vi "Read Tags.vi"(8 "error in (no error)":errorcluster, 11 "Raw Message in":refnum<class "Raw Message.lvclass">) -> (0 "error out":errorcluster, 2 "Tags":map{u32, refnum<class "Basic Type.lvclass">[]}(c390), 3 "Raw Message out":refnum<class "Raw Message.lvclass">)   [LabVIEW 2020, in "Protobuf RAW.lvlib" / "Raw Message.lvclass"]
uses:
  Raw Message.lvclass
  Tag/Basic Type.lvclass
  Raw Message.lvclass/Raw Message.ctl
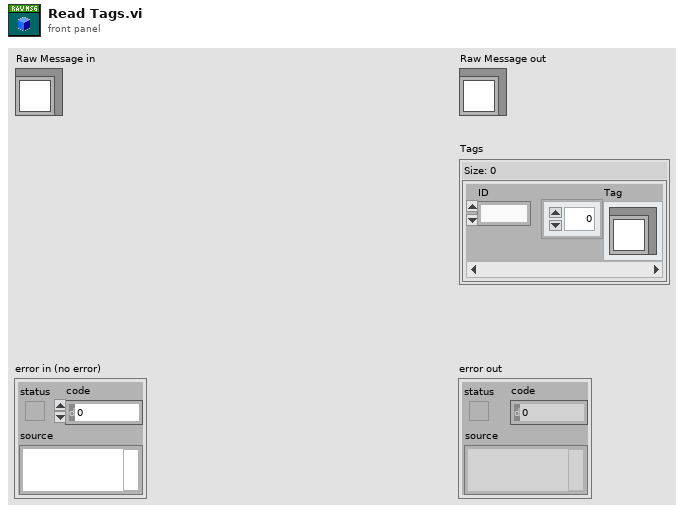
[diagram p1: front panel]
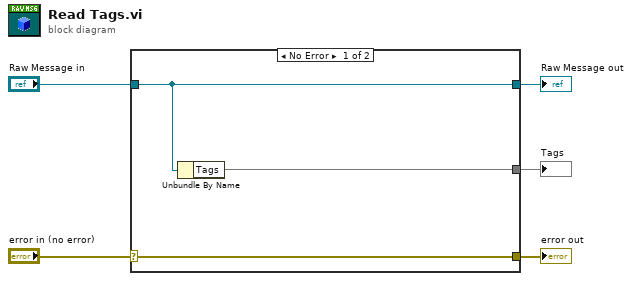
[diagram p0: block diagram]
diagram:
  n1 = case shown="No Error" "error in (no error)" {
    selector: "error in (no error)" -> [w8 w9]
    tunnel: [w8 w9] -> w4
    tunnel: [w7 w10] -> w2
    tunnel: "Raw Message in" -> [w7 w10]
    tunnel: [w6 _] -> w1
    frame No Error {
      n2 = Unbundle By Name(w7) -> ("Tags"=w6:map{u32, refnum<class "Basic Type.lvclass">[]})
    }
    frame Error {
    }
  }
  "error out" <- w4
  "Raw Message out" <- w2
  "Tags" <- w1
